vi "getShutdownEvent.vi"(11 "Controller in":refnum<class "Controller.lvclass">) -> (2 "ShutdownEvent":refnum<user-event>, 3 "Controller out":refnum<class "Controller.lvclass">)   [LabVIEW 2016]
uses:
  Controller.lvclass
  Types/ShutdownEvent.ctl
  Types/M1M3SupportTypes.lvlib
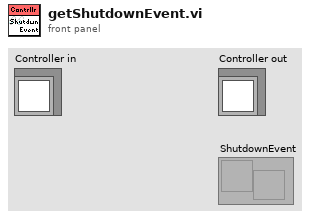
[diagram p1: front panel]
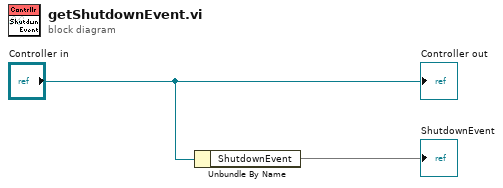
[diagram p0: block diagram]
diagram:
  n1 = Unbundle By Name("Controller in") -> ("ShutdownEvent"=→"ShutdownEvent")
  "Controller out" <- "Controller in"
